vi "mod_Interpolating FIR.vi"(5 "reset":bool, 6 "error in (no error)":errorcluster, 7 "taps":dbl[](array[numeric]), 8 "interpolation":i32, 9 "x":dbl[](array[numeric])) -> (0 "error out":errorcluster, 3 "filtered x":dbl[](array[numeric]))   [LabVIEW 2020, in "niAMT.lvlib"]
uses:
  <vilib>/addons/Modulation/niAMT.lvlib
  <vilib>/Analysis/3filter.llb/IIR Filter with I.C. (DBL).vi
  <vilib>/Analysis/NI_AALBase.lvlib
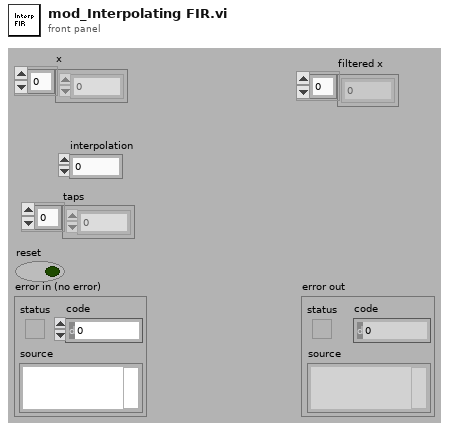
[diagram p1: front panel]
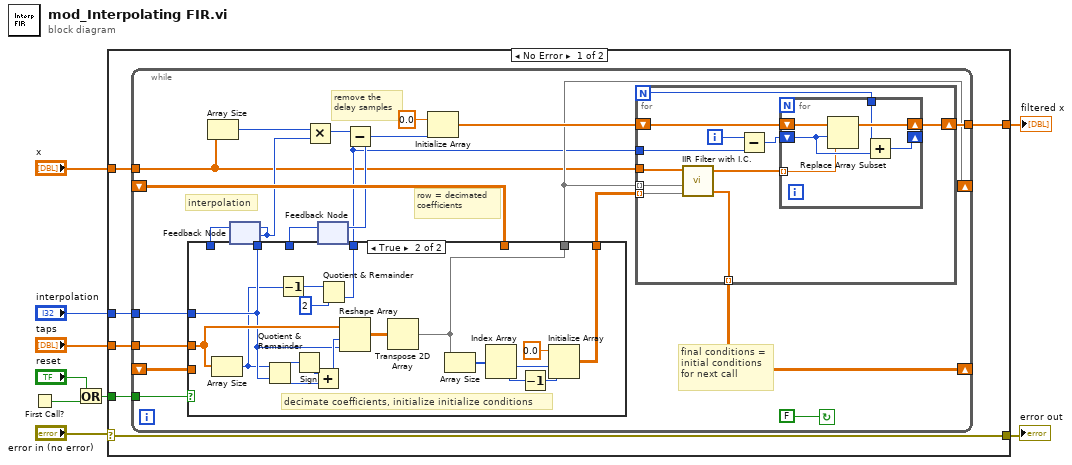
[diagram p0: block diagram]
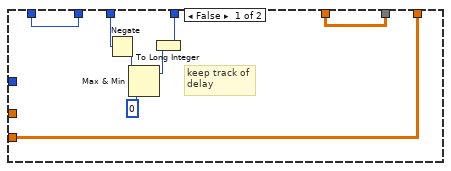
[diagram p2: hidden frame]
diagram:
  n1 = First Call?() -> (First Call?: T/F=w9:bool)
  n2 = Or(x="reset", y=w9) -> (x .or. y?=w4:bool)
  n3 = case shown="No Error" "error in (no error)" {
    selector: "error in (no error)" -> [w10 w79]
    tunnel: "x" -> [w15 _]
    tunnel: "interpolation" -> [w14 _]
    tunnel: "taps" -> [w13 _]
    tunnel: [w12 _] -> w5
    tunnel: w4 -> [w11 _]
    tunnel: [w10 w79] -> w1
    frame No Error {
      n4 = while {
        tunnel: w11 -> [w25]
        shift-right: [w20] -> _
        shift-left: _ -> [w34]
        shift-right: [w29] -> _
        shift-left: _ -> [w21]
        tunnel: w15 -> [w16]
        tunnel: w14 -> [w28]
        tunnel: w13 -> [w27]
        tunnel: [w26] -> w12
        stop <- FALSE continue-if-true
        # "remove the delay samples"
        # "row = decimated coefficients"
        # "interpolation"
        # "final conditions = initial conditions for next call"
        n5 = Array Size(array=w16) -> (size(s)=w33:i32)
        n6 = feedback #1() -> (w23:i32)  [unwired: 1 out]
        n7 = feedback #2() -> (w18:i32)  [unwired: 1 out]
        n8 = case shown="True" w25 {
          tunnel: w27 -> [_ w78]
          tunnel: w28 -> [_ w72]
          tunnel: w34 -> [w58 _]
          tunnel: [w60 w72] -> w24
          tunnel: w23 -> [w60 _]
          tunnel: [w59 w67] -> w22
          tunnel: w21 -> [w59 _]
          tunnel: [w58 w66] -> w20
          tunnel: [w53 w62] -> w17
          tunnel: w18 -> [w57 _]
          frame False {
            # "keep track of delay"
            n9 = Negate(x=w57) -> (-x=w56:i32)
            n10 = Max & Min(x=w56, y=0) -> (max(x,y)=w54:i32)  [unwired: 1 out]
            n11 = To Long Integer(number=w54) -> (32bit integer=w53:i32)
          }
          frame True {
            # "decimate coefficients, initialize initialize conditions"
            n12 = Array Size(array=w78) -> (size(s)=w65:i32)
            n13 = Quotient & Remainder(x=w65, y=w72) -> (x-y*floor(x/y)=w77:i32, floor(x/y)=w76:i32)
            n14 = Decrement(x=w65) -> (x-1=w64:i32)
            n15 = Sign(1:w77) -> (0:w75:i32)
            n16 = Add(x=w75, y=w76) -> (x+y=w73:i32)
            n17 = Quotient & Remainder(x=w64, y=2) -> (floor(x/y)=w62:i32)  [unwired: 1 out]
            n18 = Reshape Array(w78, w73, w72) -> (w74:dbl[][])
            n19 = Transpose 2D Array(2D array=w74) -> (transposed array=w66:dbl[][])
            n20 = Array Size(array=w66) -> (size(s)=w68:i32[])
            n21 = Index Array(array=w68) -> (element #1=w69:i32, element #2=w70:i32)  [unwired: 2 in]
            n22 = Decrement(x=w70) -> (x-1=w71:i32)
            n23 = Initialize Array(0.0 ("element"), w69, w71) -> (w67:dbl[][])
          }
        }
        n24 = feedback-in #1(w24) -> ()
        n25 = Multiply(x=w33, y=w24) -> (x*y=w32:i32)
        n26 = Subtract(x=w32, y=w17) -> (x-y=w19:i32)
        n27 = feedback-in #2(w19) -> ()
        n28 = Initialize Array(0.0 ("element"), w19) -> (w30:dbl[])
        n29 = for {
          N -> [w43]
          tunnel: w20 -> [w40] mode=indexing
          tunnel: w16 -> [w42]
          shift-right: [w45] -> w26
          shift-left: w30 -> [w46]
          tunnel: [w39] -> w29 mode=indexing
          tunnel: w22 -> [w38] mode=indexing
          tunnel: w17 -> [w36]
          i -> [w44]
          n30 = call-poly <vilib>:"IIR Filter with I.C..vi"("Initial X Conditions"=w38, "Forward Coefficients"=w40, "X"=w42) -> ("Final X Conditions"=w39:dbl[], "Filtered X"=w41:dbl[])  [unwired: 2 in, 4 out]
          n31 = Subtract(x=w44, y=w36) -> (x-y=w37:i32)
          n32 = for {
            shift-right: [w51] -> w45
            shift-left: w46 -> [w52]
            shift-right: [w48] -> _
            shift-left: w37 -> [w50]
            tunnel: w43 -> [w49]
            tunnel: w41 -> [w47] mode=indexing
            n33 = Replace Array Subset(array=w52, new element=w47, index=w50) -> (w51:dbl[])
            n34 = Add(x=w49, y=w50) -> (x+y=w48:i32)
          }
        }
      }
    }
    frame Error {
    }
  }
  "filtered x" <- w5
  "error out" <- w1
